vi "Build Scan Graph.vi"(8 "error in":errorcluster, 11 "Scan Driver in":refnum<class "Scan Driver.lvclass">) -> (0 "error out":errorcluster, 1 "Secondary Graph":T1, 2 "Primary Graph":T1=[{"point array"=[{"x"=401.0007, "y"=8.19568e-08}, {"x"=401.9996, "y"=4.65664e-09}, {"x"=403.0005, "y"=8.38195e-08}, {"x"=403.9992, "y"=-1.67639e-07}, {"x"=404.9998, "y"=-6.70557e-08}, {"x"=406.0002, "y"=-2.88712e-07}, {"x"=407.00059999999996, "y"=2.1793e-07}, {"x"=408.0007, "y"=3.72531e-08}, {"x"=409.0008, "y"=-6.89183e-08}, {"x"=410.0006, "y"=-1.49013e-08}]}], 3 "Scan Driver out":refnum<class "Scan Driver.lvclass">)   [LabVIEW 2009, in "Scan Driver.lvclass"]
doc: "Build and return the updated scan graph from the data store."
uses:
  Scan Driver.lvclass
  Scan Graph.ctl
  Scan Driver.lvclass/Scan Driver.ctl
  Scanners/Scanner/Scanner.lvclass
  File IO/File IO.lvclass
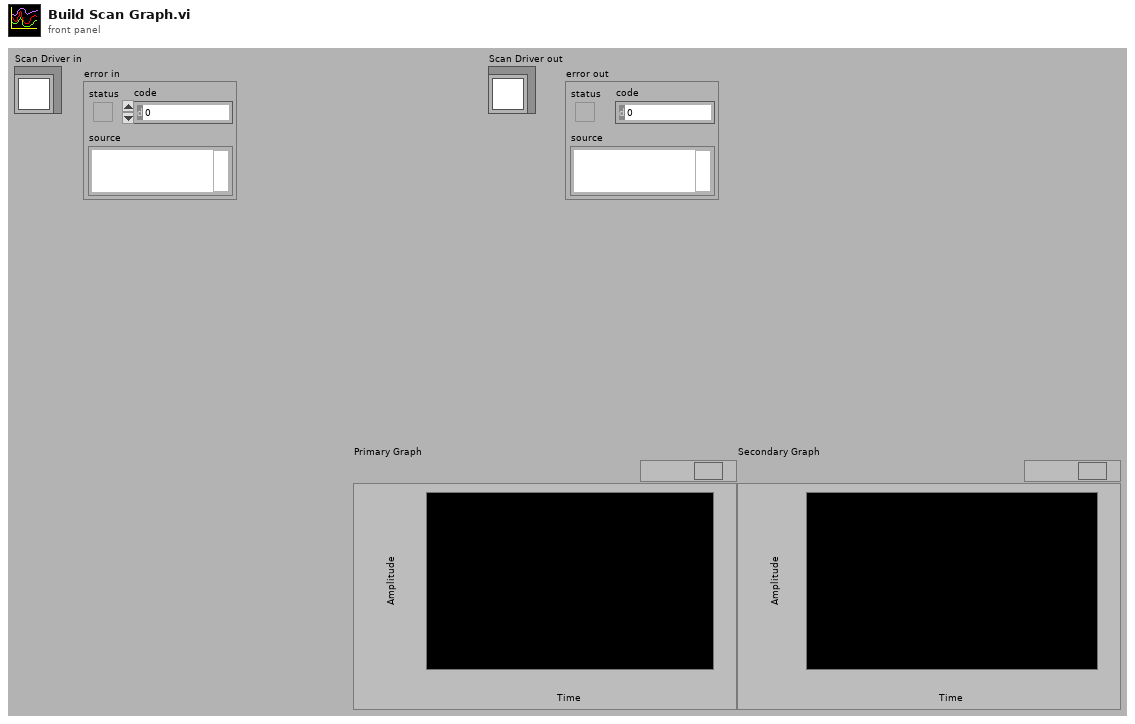
[diagram p1: front panel]
types:
  T1 = typedef "Scan Driver.lvclass/Scan Graph.ctl" = cluster{"point array":cluster{"x":dbl, "y":dbl}[]}[]
  T2 = typedef "Readable.lvclass/Data Store.ctl" = T3[][]
  T3 = typedef "Readable.lvclass/Data Point.ctl" = cluster{"t":T4, "x":T5}
  T4 = typedef "Readable.lvclass/Time.ctl" = timestamp
  T5 = typedef "Readable.lvclass/X.ctl" = dbl
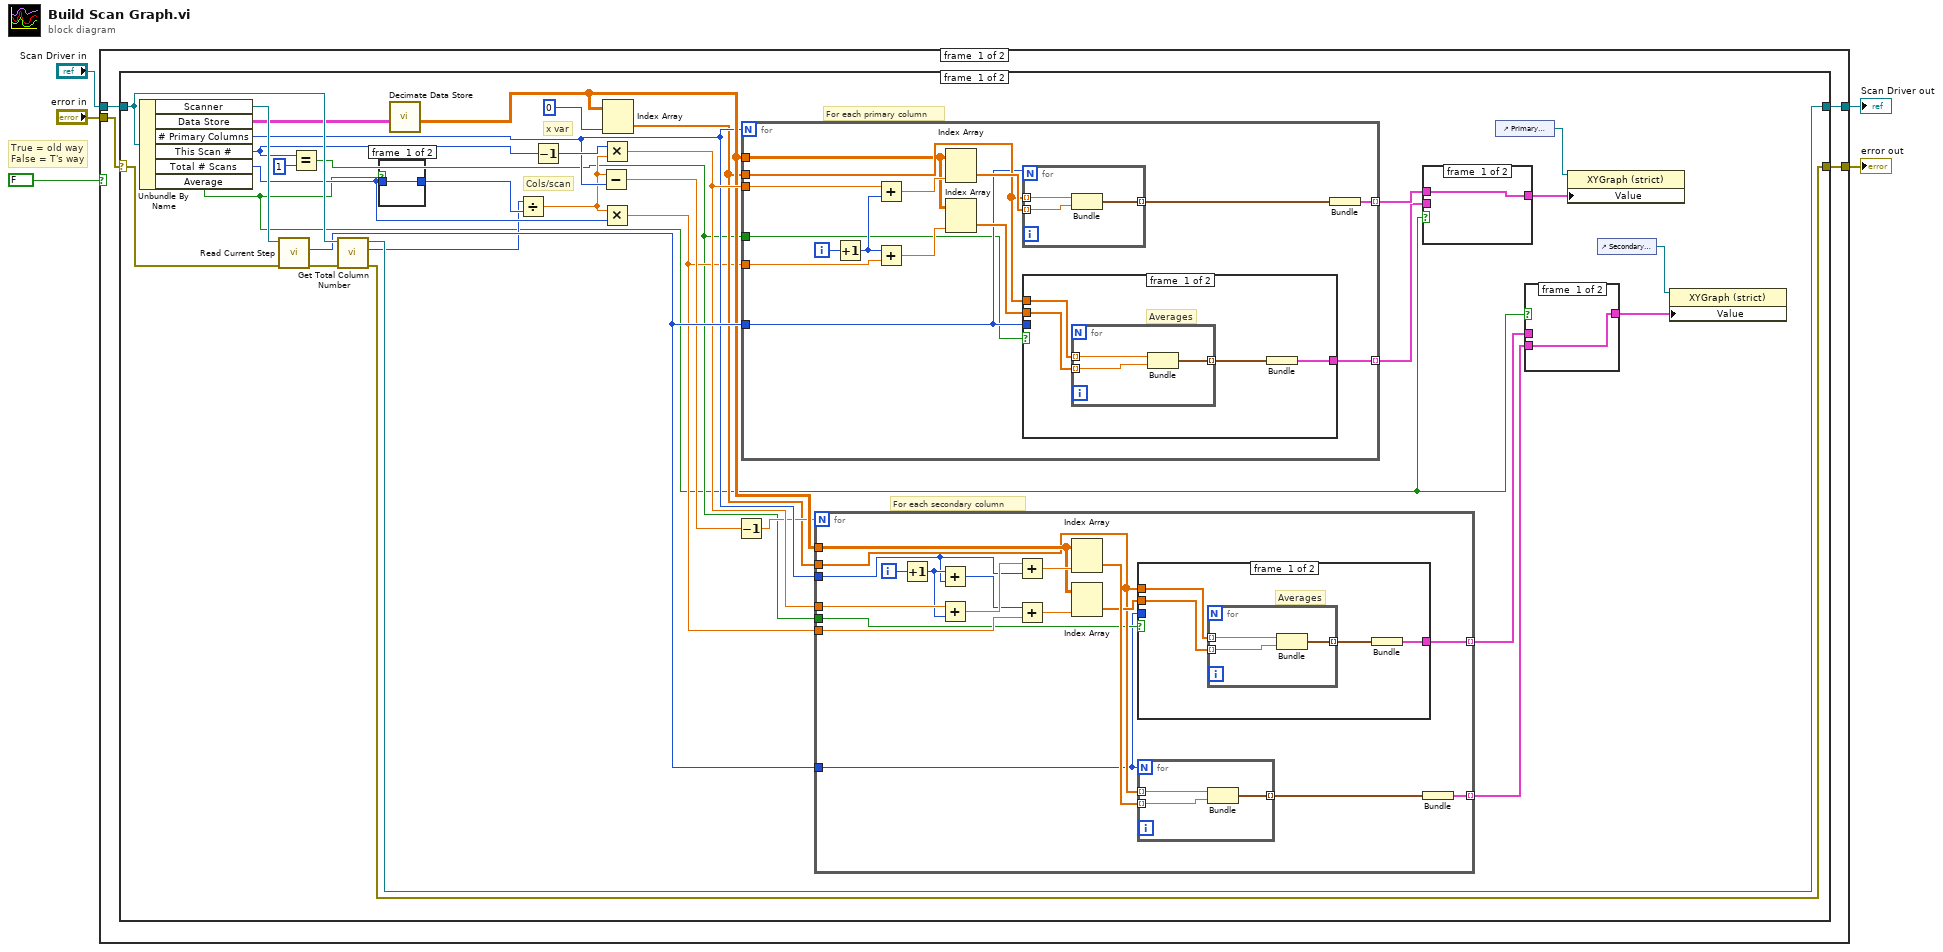
[diagram p0: block diagram]
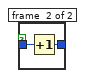
[diagram p2: hidden frame]
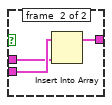
[diagram p3: hidden frame]
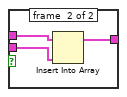
[diagram p4: hidden frame]
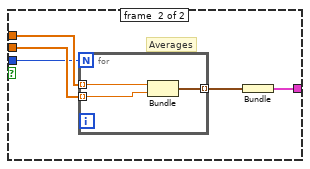
[diagram p5: hidden frame]
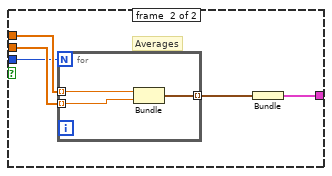
[diagram p6: hidden frame]
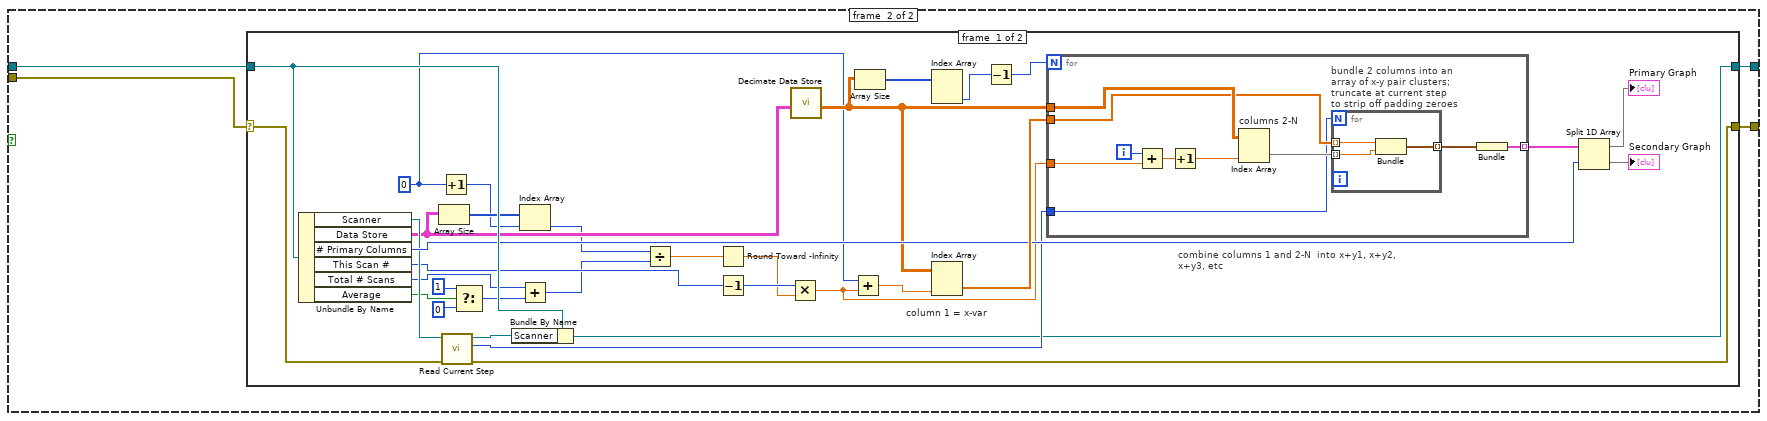
[diagram p8: hidden frame]
diagram:
  # "True = old way\nFalse = T's way"
  n1 = case shown="False" FALSE {
    tunnel: "error in" -> [w8 w128]
    tunnel: [w7 w127] -> w4
    tunnel: "Scan Driver in" -> [w9 w126]
    tunnel: [w6 w125] -> w2
    frame #0 {
      n2 = case shown="No Error" w8 {
        selector: w8 -> [w41 w124]
        tunnel: w9 -> [w40 w123]
        tunnel: [w34 w124] -> w7
        tunnel: [w36 w123] -> w6
        frame #0 {
          # "For each secondary column"
          # "For each primary column"
          # "Cols/scan"
          # "x var"
          n3 = Unbundle By Name(w40) -> ("Scanner"=w42:refnum<class "Scanner.lvclass">, "Data Store"=w38:T2, "# Primary Columns"=w25:u32, "This Scan #"=w13:u32, "Total # Scans"=w18:u32, "Average"=w10:bool)
          n4 = call-dynamic "Read Current Step.vi"("error in (no error)"=w41, "Scanner.lvclass in"=w42) -> ("error out"=w39:errorcluster, "Current Step"=w30:u32)  [unwired: 6 in, 2 out]
          n5 = Equal?(x=w13, y=1) -> (x = y?=w12:bool)
          n6 = call "Get Total Column Number.vi"("error in (no error)"=w39, "Scan Driver.lvclass"=w40) -> ("error out"=w34:errorcluster, "# of Columns"=w11:i32, "Scan Driver.lvclass"=w36:refnum<class "Scan Driver.lvclass">)  [unwired: 7 in]
          n7 = case shown="False" w10 {
            tunnel: [w43 w45] -> w35
            tunnel: w18 -> [w43 w44]
            frame #0 {
            }
            frame #1 {
              n8 = Increment(x=w44) -> (x+1=w45:u32)
            }
          }
          n9 = call "Decimate Data Store.vi"("Data Store"=w38) -> ("Data Points"=w27:T5[][])  [unwired: 9 in, 1 out]
          n10 = Divide(x=w11, y=w35) -> (x/y=w22:dbl)
          n11 = Decrement(x=w13) -> (x-1=w31:u32)
          n12 = Subtract(x=w22, y=w25) -> (x-y=w26:dbl)
          n13 = Multiply(x=w31, y=w22) -> (x*y=w28:dbl)
          n14 = Multiply(x=w22, y=w18) -> (x*y=w17:dbl)
          n15 = Index Array(array=w27, index (col)=0) -> (element=w23:T5[])  [unwired: 1 in]
          n16 = Decrement(x=w26) -> (x-1=w24:dbl)
          n17 = for {
            N: w25 -> [_]
            tunnel: w27 -> [w98]
            tunnel: w23 -> [w99]
            tunnel: w28 -> [w103]
            tunnel: [w93] -> w20 mode=indexing
            tunnel: w30 -> [w91]
            tunnel: w17 -> [w96]
            tunnel: [w92] -> w19 mode=indexing
            tunnel: w12 -> [w90]
            i -> [w104]
            n18 = Increment(x=w104) -> (x+1=w97:i32)
            n19 = Add(x=w103, y=w97) -> (x+y=w100:dbl)
            n20 = Add(x=w97, y=w96) -> (x+y=w95:dbl)
            n21 = Index Array(array=w98, index (col)=w100) -> (element=w102:T5[])  [unwired: 1 in]
            n22 = Index Array(array=w98, index (col)=w95) -> (element=w94:T5[])  [unwired: 1 in]
            n23 = for {
              N: w91 -> [_]
              tunnel: w99 -> [w122] mode=indexing
              tunnel: w102 -> [w121] mode=indexing
              tunnel: [w120] -> w101 mode=indexing
              n24 = Bundle("x"=w122, "x"=w121) -> (w120:cluster{"x":T5, "x":T5})  [unwired: 1 in]
            }
            n25 = case shown="False" w90 {
              tunnel: w99 -> [w107 w116]
              tunnel: w94 -> [w106 w115]
              tunnel: [w105 w113] -> w92
              tunnel: w91 -> [_ w112]
              frame #0 {
                # "Averages"
                n26 = for {
                  tunnel: w107 -> [w111] mode=indexing
                  tunnel: w106 -> [w110] mode=indexing
                  tunnel: [w109] -> w108 mode=indexing
                  n27 = Bundle("x"=w111, "x"=w110) -> (w109:cluster{"x":T5, "x":T5})  [unwired: 1 in]
                }
                n28 = Bundle(w108) -> (w105:cluster{cluster{"x":T5, "x":T5}[]})  [unwired: 1 in]
              }
              frame #1 {
                # "Averages"
                n29 = for {
                  N: w112 -> [_]
                  tunnel: w116 -> [w119] mode=indexing
                  tunnel: w115 -> [w118] mode=indexing
                  tunnel: [w117] -> w114 mode=indexing
                  n30 = Bundle("x"=w119, "x"=w118) -> (w117:cluster{"x":T5, "x":T5})  [unwired: 1 in]
                }
                n31 = Bundle(w114) -> (w113:cluster{cluster{"x":T5, "x":T5}[]})  [unwired: 1 in]
              }
            }
            n32 = Bundle(w101) -> (w93:cluster{cluster{"x":T5, "x":T5}[]})  [unwired: 1 in]
          }
          n33 = for {
            N: w24 -> [_]
            tunnel: w27 -> [w61]
            tunnel: w23 -> [w60]
            tunnel: w28 -> [w70]
            tunnel: [w66] -> w29 mode=indexing
            tunnel: w30 -> [w54]
            tunnel: w25 -> [w56]
            tunnel: w17 -> [w62]
            tunnel: [w59] -> w15 mode=indexing
            tunnel: w12 -> [w55]
            i -> [w71]
            n34 = Increment(x=w71) -> (x+1=w58:i32)
            n35 = Add(x=w58, y=w56) -> (x+y=w57:u32)
            n36 = Add(x=w70, y=w58) -> (x+y=w67:dbl)
            n37 = Add(x=w67, y=w56) -> (x+y=w65:dbl)
            n38 = Add(x=w57, y=w62) -> (x+y=w64:dbl)
            n39 = Index Array(array=w61, index (col)=w65) -> (element=w69:T5[])  [unwired: 1 in]
            n40 = Index Array(array=w61, index (col)=w64) -> (element=w63:T5[])  [unwired: 1 in]
            n41 = case shown="False" w55 {
              tunnel: w63 -> [w72 w83]
              tunnel: w60 -> [w73 w81]
              tunnel: [w74 w80] -> w59
              tunnel: w54 -> [_ w79]
              frame #0 {
                # "Averages"
                n42 = for {
                  tunnel: w72 -> [w78] mode=indexing
                  tunnel: [w77] -> w75 mode=indexing
                  tunnel: w73 -> [w76] mode=indexing
                  n43 = Bundle("x"=w76, "x"=w78) -> (w77:cluster{"x":T5, "x":T5})  [unwired: 1 in]
                }
                n44 = Bundle(w75) -> (w74:cluster{cluster{"x":T5, "x":T5}[]})  [unwired: 1 in]
              }
              frame #1 {
                # "Averages"
                n45 = for {
                  N: w79 -> [_]
                  tunnel: w83 -> [w86] mode=indexing
                  tunnel: [w85] -> w82 mode=indexing
                  tunnel: w81 -> [w84] mode=indexing
                  n46 = Bundle("x"=w84, "x"=w86) -> (w85:cluster{"x":T5, "x":T5})  [unwired: 1 in]
                }
                n47 = Bundle(w82) -> (w80:cluster{cluster{"x":T5, "x":T5}[]})  [unwired: 1 in]
              }
            }
            n48 = for {
              N: w54 -> [_]
              tunnel: w60 -> [w89] mode=indexing
              tunnel: w69 -> [w88] mode=indexing
              tunnel: [w87] -> w68 mode=indexing
              n49 = Bundle("x"=w89, "x"=w88) -> (w87:cluster{"x":T5, "x":T5})  [unwired: 1 in]
            }
            n50 = Bundle(w68) -> (w66:cluster{cluster{"x":T5, "x":T5}[]})  [unwired: 1 in]
          }
          n51 = case shown="False" w10 {
            tunnel: [w50 w53] -> w21
            tunnel: w20 -> [w50 w52]
            tunnel: w19 -> [_ w51]
            frame #0 {
            }
            frame #1 {
              n52 = Insert Into Array(array=w52, new element=w51) -> (w53:cluster{cluster{"x":T5, "x":T5}[]}[])  [unwired: 1 in]
            }
          }
          n53 = control-ref of="Primary Graph"() -> (w32:refnum<vi>)
          n54 = case shown="False" w10 {
            tunnel: w29 -> [w46 w49]
            tunnel: [w46 w48] -> w16
            tunnel: w15 -> [_ w47]
            frame #0 {
            }
            frame #1 {
              n55 = Insert Into Array(array=w49, new element=w47) -> (w48:cluster{cluster{"x":T5, "x":T5}[]}[])  [unwired: 1 in]
            }
          }
          n56 = property class="XYGraph (strict)"(reference=w32, "Value"=w21) -> ()  [unwired: 1 in, 2 out]
          n57 = control-ref of="Secondary Graph"() -> (w33:refnum<vi>)
          n58 = property class="XYGraph (strict)"(reference=w33, "Value"=w16) -> ()  [unwired: 1 in, 2 out]
        }
        frame #1 {
        }
      }
    }
    frame #1 {
      n59 = case shown="No Error" w128 {
        selector: w128 -> [w161 w176]
        tunnel: [w151 w176] -> w127
        tunnel: w126 -> [w153 w175]
        tunnel: [w148 w175] -> w125
        frame #0 {
          w141 = 0
          n60 = Unbundle By Name(w153) -> ("Scanner"=w149:refnum<class "Scanner.lvclass">, "Data Store"=w144:T2, "# Primary Columns"=w152:u32, "This Scan #"=w138:u32, "Total # Scans"=w139:u32, "Average"=w133:bool)
          n61 = Array Size(array=w144) -> (size(s)=w143:i32[])
          n62 = Increment(x=w141) -> (x+1=w136:i32)
          n63 = call-dynamic "Read Current Step.vi"("error in (no error)"=w161, "Scanner.lvclass in"=w149) -> ("error out"=w151:errorcluster, "Current Step"=w150:u32, "Scanner.lvclass out"=w147:refnum<class "Scanner.lvclass">)  [unwired: 6 in, 1 out]
          n64 = Select(t=1, s=w133, f=0) -> (s? t:f=w131:i32)
          n65 = Bundle By Name(cluster=w153, "Scanner"=w147) -> (w148:refnum<class "Scan Driver.lvclass">)
          n66 = Index Array(array=w143, index=w136) -> (element=w142:i32)
          n67 = Add(x=w139, y=w131) -> (x+y=w132:u32)
          n68 = Divide(x=w142, y=w132) -> (x/y=w140:dbl)
          n69 = Round Toward -Infinity(1:w140) -> (0:w134:dbl)
          n70 = Decrement(x=w138) -> (x-1=w135:u32)
          n71 = Multiply(x=w135, y=w134) -> (x*y=w137:dbl)
          n72 = call "Decimate Data Store.vi"("Data Store"=w144) -> ("Data Points"=w146:T5[][])  [unwired: 9 in, 1 out]
          n73 = Add(x=w141, y=w137) -> (x+y=w145:dbl)
          n74 = Array Size(array=w146) -> (size(s)=w157:i32[])
          n75 = Index Array(array=w157) -> (element #2=w154:i32)  [unwired: 2 in, 1 out]
          n76 = Index Array "column 1 = x-var"(array=w146, index (col)=w145) -> (element=w158:T5[])  [unwired: 1 in]
          n77 = Decrement(x=w154) -> (x-1=w156:i32)
          n78 = for "combine columns 1 and 2-N  into x+y1, x+y2, x+y3, etc" {
            N: w156 -> [_]
            tunnel: w158 -> [w167]
            tunnel: w146 -> [w171]
            tunnel: [w166] -> w155 mode=indexing
            tunnel: w150 -> [w164]
            tunnel: w137 -> [w162]
            i -> [w170]
            n79 = Add(x=w170, y=w162) -> (x+y=w163:dbl)
            n80 = Increment(x=w163) -> (x+1=w169:dbl)
            n81 = Index Array "columns 2-N"(array=w171, index (col)=w169) -> (element=w168:T5[])  [unwired: 1 in]
            n82 = for "bundle 2 columns into an\narray of x-y pair clusters;\ntruncate at current step\nto strip off padding zeroes" {
              N: w164 -> [_]
              tunnel: w168 -> [w173] mode=indexing
              tunnel: w167 -> [w174] mode=indexing
              tunnel: [w172] -> w165 mode=indexing
              n83 = Bundle("x"=w174, "x"=w173) -> (w172:cluster{"x":T5, "x":T5})  [unwired: 1 out]
            }
            n84 = Bundle(w165) -> (w166:cluster{cluster{"x":T5, "x":T5}[]})  [unwired: 1 in]
          }
          n85 = Split 1D Array(array=w155, index=w152) -> (first subarray=→"Primary Graph":cluster{cluster{"x":T5, "x":T5}[]}[], second subarray=→"Secondary Graph":cluster{cluster{"x":T5, "x":T5}[]}[])
        }
        frame #1 {
        }
      }
    }
  }
  "error out" <- w4
  "Scan Driver out" <- w2
